vi "Controller Open Synchronization Objects.vi"(8 "error in (no error)":errorcluster, 11 "FOFB Configuration":T4={"FOFB Parameters"={"Network"={"FOFB Controller IP"="", "LNLS Control Network IP"="", "LNLS Control Network Power Supplies TCP Port"=0, "LNLS Control Network FOFB Configuration TCP Port"=0, "LNLS Control Network BPMs TCP Port"=0, "Monitoring Data TCP Port"=0, "Fast Archiver TCP Port"=0, "Fast Command TCP Port"=0, "TCP Listening Timeout"=0}, "Fast Acquisition"={"Sampling Period"=0, "Data Buffer Size"=0, "Monitoring Period"=0}, "Acquisition Network"=[], "Actuation Network"=[]}, "Number of Acquisition Chassis"=0, "Number of Actuation Chassis"=0, "Number of BPM Readings"=0, "BPM Reading Names"=[], "Selected BPM Readings"=[0, 1, 2, 3, 4, 5, 6, 7, 8, 9, 10, 11, 12, 13, 14, 15, 16, 17, 18, 19, 20, 21, 22, 23, 24, 25, 26, 27, 28, 29, 30, 31, 32, 33, 34, 35, 36, 37, 38, 39, 40, 41, 42, 43, 44, 45, 46, 47, 48, 49], "Number of Correctors"=0, "Corrector Names"=[], "Selected Correctors"=[0, 1, 2, 3, 4, 5, 6, 7, 8, 9, 10, 11, 12, 13, 14, 15, 16, 17, 18, 19, 20, 21, 22, 23, 24, 25, 26, 27, 28, 29, 30, 31, 32, 33, 34, 35, 36, 37, 38, 39, 40, 41, 42, 43, 44, 45, 46, 47, 48, 49], "Response Matrix"=[], "Reference Orbit"=[], "Correction Matrix"=[], "FPGA Filter Sets"=[], "Acquisition Chassis Names"=[], "Actuation Chassis Names"=[], "Acquisition Variables"=[], "Actuation Variables"=[], "PS Matrix Mapping"=[], "Inverse PS Matrix Mapping"=[], "BPM Matrix Mapping"=[], "Inverse BPM Matrix Mapping"=[], "BPM Planes"=[], "Corrector Planes"=[]}) -> (0 "error out":errorcluster, 3 "Sync Objects":T1)   [LabVIEW 2011, in "Controller VIs.lvlib"]
uses:
  Controller VIs.lvlib
  Types Definitions/Type FOFB Configuration.ctl
  Types Definitions/Type FOFB Parameters.ctl
  Types Definitions/Type Network Configuration.ctl
  Types Definitions/Type FA Configuration.ctl
  Types Definitions/Type Acquisition Network Configuration.ctl
  Types Definitions/Type Actuation Network Configuration.ctl
  Types Definitions/Type Synchronization Objects.ctl
  Types Definitions/Type Blocking Synchronization Objects.ctl
  Types Definitions/Type Monitoring Data.ctl
  Types Definitions/Type Operation Mode State.ctl
  Types Definitions/Type Diagnostics Data.ctl
  Types Definitions/Type CPU Loads Array.ctl
  Types Definitions/Type CPU Loads.ctl
  Types Definitions/Type Non-blocking Synchronization Objects.ctl
  Types Definitions/Type FOFB Variables.ctl
  Types Definitions/Type Actuation State.ctl
  Type Definitions.lvlib
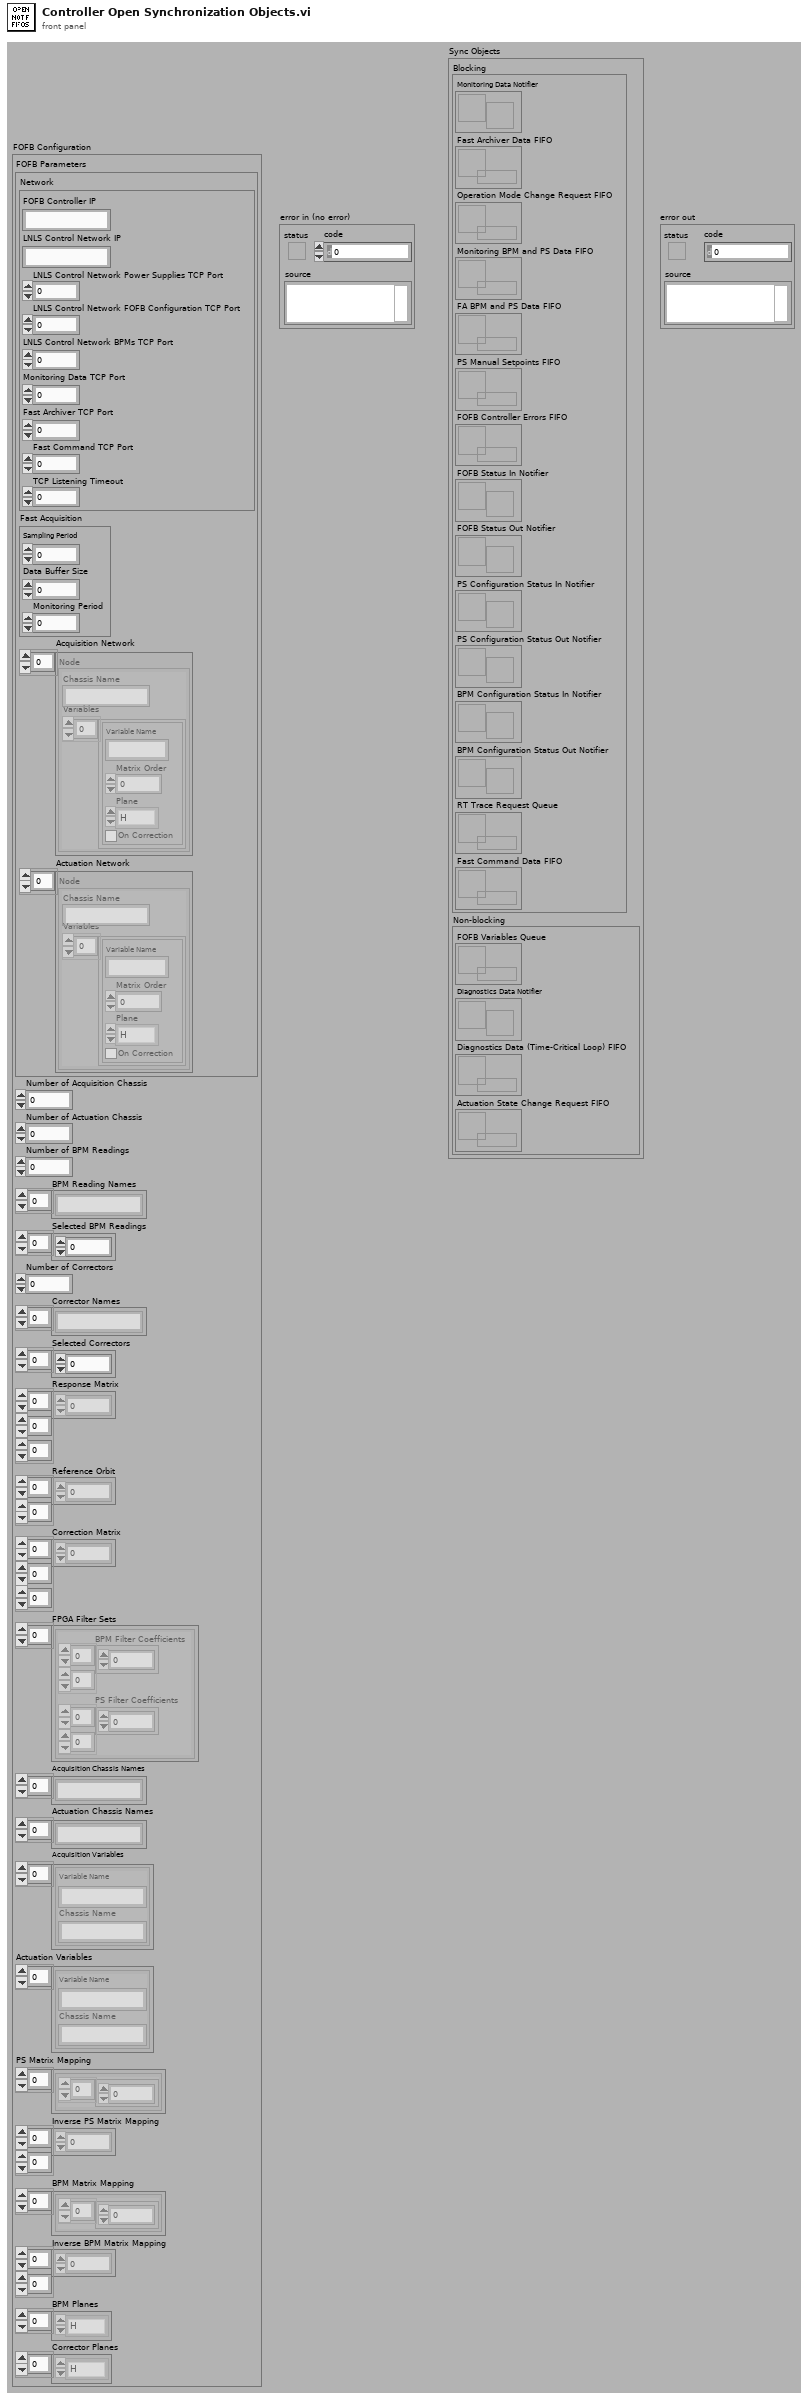
[diagram p1: front panel]
types:
  T1 = typedef "Type Definitions.lvlib/Type Synchronization Objects.ctl" = cluster{"Blocking":T2, "Non-blocking":T3}
  T2 = typedef "Type Definitions.lvlib/Type Blocking Synchronization Objects.ctl" = cluster{"Monitoring Data Notifier":refnum<notifier>, "Fast Archiver Data FIFO":refnum<queue>, "Operation Mode Change Request FIFO":refnum<k33>, "Monitoring BPM and PS Data FIFO":refnum<k33>, "FA BPM and PS Data FIFO":refnum<k33>, "PS Manual Setpoints FIFO":refnum<k33>, "FOFB Controller Errors FIFO ":refnum<k33>, "FOFB Status In Notifier":refnum<notifier>, "FOFB Status Out Notifier":refnum<notifier>, "PS Configuration Status In Notifier":refnum<notifier>, "PS Configuration Status Out Notifier":refnum<notifier>, "BPM Configuration Status In Notifier":refnum<notifier>, "BPM Configuration Status Out Notifier":refnum<notifier>, "RT Trace Request Queue":refnum<queue>, "Fast Command Data FIFO":refnum<k33>}
  T3 = typedef "Type Definitions.lvlib/Type Non-blocking Synchronization Objects.ctl" = cluster{"FOFB Variables Queue":refnum<queue>, "Diagnostics Data Notifier":refnum<notifier>, "Diagnostics Data (Time-Critical Loop) FIFO":refnum<k33>, "Actuation State Change Request FIFO":refnum<k33>}
  T4 = typedef "Type Definitions.lvlib/Type FOFB Configuration.ctl" = cluster{"FOFB Parameters":T5, "Number of Acquisition Chassis":i32, "Number of Actuation Chassis":i32, "Number of BPM Readings":i32, "BPM Reading Names":string[], "Selected BPM Readings":u32[], "Number of Correctors":i32, "Corrector Names":string[], "Selected Correctors":u32[], "Response Matrix":dbl[][][], "Reference Orbit":dbl[][], "Correction Matrix":dbl[][][], "FPGA Filter Sets":cluster{"BPM Filter Coefficients":dbl[][], "PS Filter Coefficients":dbl[][]}[], "Acquisition Chassis Names":string[], "Actuation Chassis Names":string[], "Acquisition Variables":cluster{"Variable Name":string, "Chassis Name":string}[], "Actuation Variables":cluster{"Variable Name":string, "Chassis Name":string}[], "PS Matrix Mapping":cluster{u32[]}[], "Inverse PS Matrix Mapping":u32[][], "BPM Matrix Mapping":cluster{u32[]}[], "Inverse BPM Matrix Mapping":u32[][], "BPM Planes":enum8{"H", "V"}[], "Corrector Planes":enum8{"H", "V"}[]}
  T5 = typedef "Type Definitions.lvlib/Type FOFB Parameters.ctl" = cluster{"Network":T6, "Fast Acquisition":T7, "Acquisition Network":T8, "Actuation Network":T9}
  T6 = typedef "Type Definitions.lvlib/Type Network Configuration.ctl" = cluster{"FOFB Controller IP":string, "LNLS Control Network IP":string, "LNLS Control Network Power Supplies TCP Port":u16, "LNLS Control Network FOFB Configuration TCP Port":u16, "LNLS Control Network BPMs TCP Port":u16, "Monitoring Data TCP Port":u16, "Fast Archiver TCP Port":u16, "Fast Command TCP Port":u16, "TCP Listening Timeout":i32}
  T7 = typedef "Type Definitions.lvlib/Type FA Configuration.ctl" = cluster{"Sampling Period":u32, "Data Buffer Size":u32, "Monitoring Period":u32}
  T8 = typedef "Type Definitions.lvlib/Type Acquisition Network Configuration.ctl" = cluster{"Chassis Name":string, "Variables":cluster{"Variable Name":string, "Matrix Order":u32, "Plane":enum8{"H", "V"}, "On Correction":bool}[]}[]
  T9 = typedef "Type Definitions.lvlib/Type Actuation Network Configuration.ctl" = cluster{"Chassis Name":string, "Variables":cluster{"Variable Name":string, "Matrix Order":u32, "Plane":enum8{"H", "V"}, "On Correction":bool}[]}[]
  T10 = typedef "Type Definitions.lvlib/Type Operation Mode State.ctl" = enum8{"Idle Mode", "Manual Mode", "FOFB Mode"}
  T11 = typedef "Type Definitions.lvlib/Type FOFB Variables.ctl" = cluster{"Reference Orbit":dbl[], "Response Matrix":dbl[][], "Correction Matrix":dbl[][], "FPGA Filter":cluster{"BPM Filter Coefficients":dbl[][], "PS Filter Coefficients":dbl[][]}, "Selected BPM Readings":u32[], "Selected Correctors":u32[], "BPM Planes":enum8{"H", "V"}[], "Corrector Planes":enum8{"H", "V"}[], "Fast Command Enabled":bool, "Horizontal Gain":dbl, "Vertical Gain":dbl, "Horizontal Distortion Threshold":dbl, "Vertical Distortion Threshold":dbl}
  T12 = cluster{"read mode":enum16{"polling", "blocking"}, "write mode":enum16{"polling", "blocking"}}
  T13 = typedef "Type Definitions.lvlib/Type Diagnostics Data.ctl" = cluster{"Time-Critical Loop Missed Iterations":u32, "Time-Critical Loop Execution Time (usec)":u32, "Available Memory (bytes)":u32, "CPU Loads Array":T14}
  T14 = typedef "Type Definitions.lvlib/Type CPU Loads Array.ctl" = T15[]
  T15 = typedef "Type Definitions.lvlib/Type CPU Loads.ctl" = cluster{"Total (%)":dbl, "Time Critical (%)":dbl, "Timed Structures (%)":dbl, "High (%)":dbl, "Above Normal (%)":dbl, "Normal (%)":dbl, "Background (%)":dbl, "Idle (%)":dbl, "ISR (%)":dbl}
  T16 = typedef "Type Definitions.lvlib/Type Monitoring Data.ctl" = cluster{"Timestamp":timestamp, "BPM Readings":dbl[], "PS Readings":dbl[], "PS FOFB Setpoints":dbl[], "PS Status per Rack":u8[], "PS ON-OFF per Rack":u8[], "Operation Mode":T10, "Diagnostics Data":T13, "Controller Status Table":i32[]}
  T17 = typedef "Type Definitions.lvlib/Type Actuation State.ctl" = enum8{"Only reading", "Manual", "FOFB Initialization", "FOFB", "FOFB Stopping"}
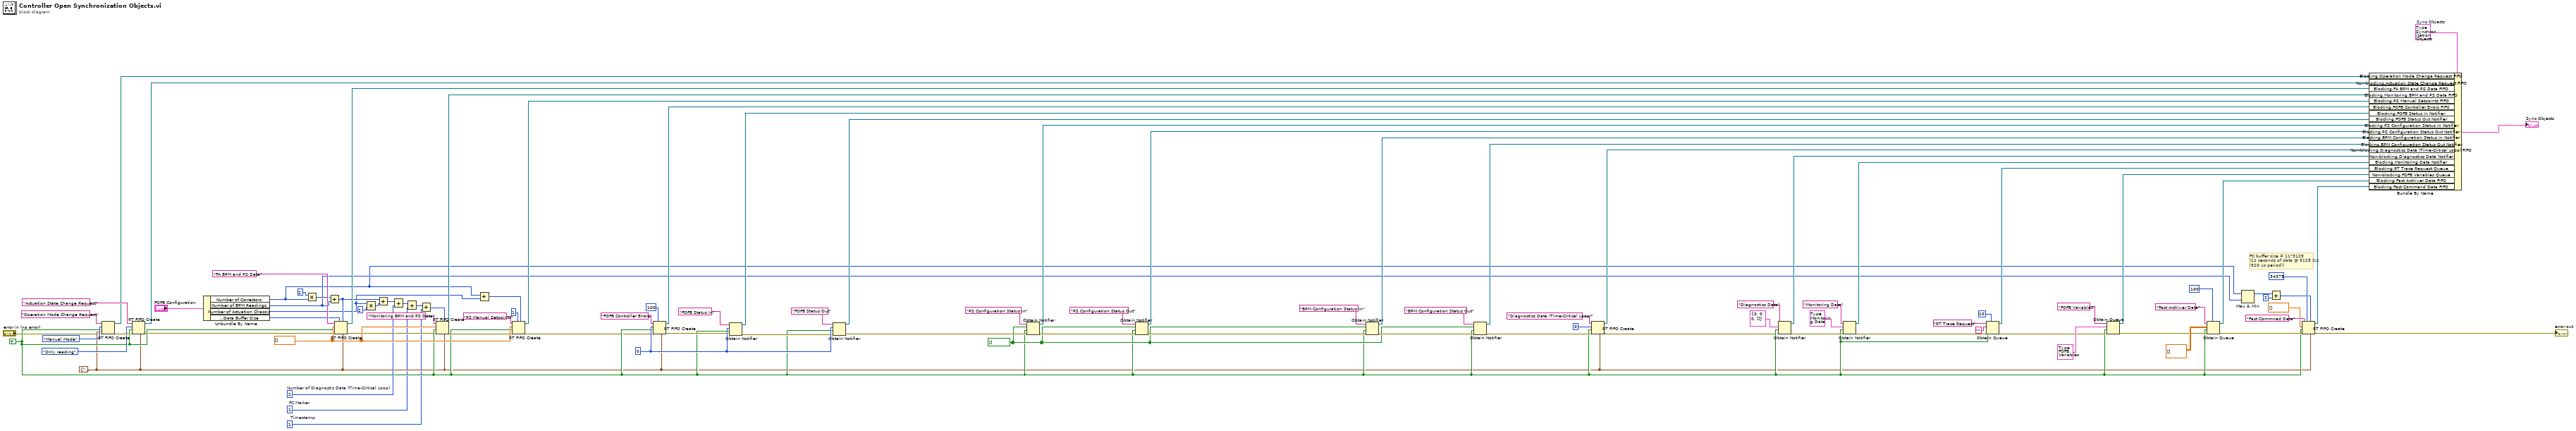
[diagram p0: block diagram]
diagram:
  w5 = 1  # FC Marker
  w4 = 1  # Timestamp
  w30 = bool[] []
  w64 = 2  # Number of Diagnostic Data (Time-Critical Loop)
  w14 = T12 {"read mode"=enum."blocking", "write mode"=enum."blocking"} ("r/w modes (polling,polling)")
  w41 = u16 0 ("elements in array (1)")
  w97 = T1 {"Blocking"={"Monitoring Data Notifier"=refnum, "Fast Archiver Data FIFO"=refnum, "Operation Mode Change Request FIFO"=refnum, "Monitoring BPM and PS Data FIFO"=refnum, "FA BPM and PS Data FIFO"=refnum, "PS Manual Setpoints FIFO"=refnum, "FOFB Controller Errors FIFO "=refnum, "FOFB Status In Notifier"=refnum, "FOFB Status Out Notifier"=refnum, "PS Configuration Status In Notifier"=refnum, "PS Configuration Status Out Notifier"=refnum, "BPM Configuration Status In Notifier"=refnum, "BPM Configuration Status Out Notifier"=refnum, "RT Trace Request Queue"=refnum, "Fast Command Data FIFO"=refnum}, "Non-blocking"={"FOFB Variables Queue"=refnum, "Diagnostics Data Notifier"=refnum, "Diagnostics Data (Time-Critical Loop) FIFO"=refnum, "Actuation State Change Request FIFO"=refnum}}  # Sync Objects
  w20 = TRUE
  w74 = dbl[] [] ("BPM Readings")
  # "FC buffer size = 11*3125\n(11 seconds of data @ 3125 S/s\n(320 us period))"
  n1 = RT FIFO Create(0:"Operation Mode Change Request" ("name (unnamed)"), 1:Type_Operation_Mode_State."Manual Mode" ("Operation Mode"), 2:w20, 3:"error in (no error)", 7:w14) -> (8:w54:refnum<k33>, 11:w94:errorcluster)  [unwired: 3 in, 1 out]
  n2 = RT FIFO Create(0:"Actuation State Change Request" ("name (unnamed)"), 1:Type_Actuation_State."Only reading" ("Actuation State"), 2:w20, 3:w94, 7:w14) -> (8:w89:refnum<k33>, 11:w9:errorcluster)  [unwired: 3 in, 1 out]
  n3 = Unbundle By Name("FOFB Configuration") -> ("Number of Correctors"=w19:i32, "Number of BPM Readings"=w21:i32, "Number of Actuation Chassis"=w18:i32, "FOFB Parameters.Fast Acquisition.Data Buffer Size"=w84:u32)
  n4 = Multiply(x=2 ("y"), y=w19) -> (x*y=w85:i32)
  n5 = Add(x=w85, y=w21) -> (x+y=w78:i32)
  n6 = RT FIFO Create(0:"FA BPM and PS Data" ("name (unnamed)"), 1:w74, 2:w20, 3:w9, 4:w84, 6:w78, 7:w14) -> (8:w98:refnum<k33>, 11:w10:errorcluster)  [unwired: 1 in, 1 out]
  n7 = Multiply(x=w18, y=2) -> (x*y=w70:i32)
  n8 = Add(x=w78, y=w70) -> (x+y=w65:i32)
  n9 = Add(x=w65, y=w64) -> (x+y=w7:i32)
  n10 = Add(x=w7, y=w5) -> (x+y=w6:i32)
  n11 = Add(x=w6, y=w4) -> (x+y=w8:i32)
  n12 = RT FIFO Create(0:"Monitoring BPM and PS Data" ("name (unnamed)"), 1:w74, 2:w20, 3:w10, 6:w8, 7:w14) -> (8:w87:refnum<k33>, 11:w73:errorcluster)  [unwired: 2 in, 1 out]
  n13 = Add(x=w19, y=w18) -> (x+y=w72:i32)
  n14 = RT FIFO Create(0:"PS Manual Setpoints" ("name (unnamed)"), 1:w74, 2:w20, 3:w73, 4:u32 1 ("size (10)"), 6:w72) -> (8:w71:refnum<k33>, 11:w13:errorcluster)  [unwired: 2 in, 1 out]
  n15 = RT FIFO Create(0:"FOFB Controller Errors" ("name (unnamed)"), 1:w41, 2:w20, 3:w13, 4:u32 100 ("elements in array (1)"), 7:w14) -> (8:w52:refnum<k33>, 11:w38:errorcluster)  [unwired: 2 in, 1 out]
  n16 = Obtain Notifier(name (unnamed)="FOFB Status In", notification data type=w41, create if not found? (T)=w20, error in (no error)=w38) -> (notifier out=w39:refnum<notifier>, error out=w37:errorcluster)  [unwired: 1 out]
  n17 = Obtain Notifier(name (unnamed)="FOFB Status Out", notification data type=w41, create if not found? (T)=w20, error in (no error)=w37) -> (notifier out=w40:refnum<notifier>, error out=w32:errorcluster)  [unwired: 1 out]
  n18 = Obtain Notifier(name (unnamed)="PS Configuration Status In", notification data type=w30, create if not found? (T)=w20, error in (no error)=w32) -> (notifier out=w36:refnum<notifier>, error out=w50:errorcluster)  [unwired: 1 out]
  n19 = Obtain Notifier(name (unnamed)="PS Configuration Status Out", notification data type=w30, create if not found? (T)=w20, error in (no error)=w50) -> (notifier out=w35:refnum<notifier>, error out=w31:errorcluster)  [unwired: 1 out]
  n20 = Obtain Notifier(name (unnamed)="BPM Configuration Status In", notification data type=w30, create if not found? (T)=w20, error in (no error)=w31) -> (notifier out=w34:refnum<notifier>, error out=w45:errorcluster)  [unwired: 1 out]
  n21 = Obtain Notifier(name (unnamed)="BPM Configuration Status Out", notification data type=w30, create if not found? (T)=w20, error in (no error)=w45) -> (notifier out=w33:refnum<notifier>, error out=w44:errorcluster)  [unwired: 1 out]
  n22 = RT FIFO Create(0:"Diagnostics Data (Time-Critical Loop)" ("name (unnamed)"), 1:u32 0 ("elements in array (1)"), 2:w20, 3:w44, 7:w14) -> (8:w66:refnum<k33>, 11:w12:errorcluster)  [unwired: 3 in, 1 out]
  n23 = Obtain Notifier(name (unnamed)="Diagnostics Data", notification data type=T13 {"Time-Critical Loop Missed Iterations"=0, "Time-Critical Loop Execution Time (usec)"=0, "Available Memory (bytes)"=0, "CPU Loads Array"=[]} ("Diagnostics Data"), create if not found? (T)=w20, error in (no error)=w12) -> (notifier out=w79:refnum<notifier>, error out=w80:errorcluster)  [unwired: 1 out]
  n24 = Obtain Notifier(name (unnamed)="Monitoring Data", notification data type=T16 {"Timestamp"=timestamp(0 s since 1904-01-01), "BPM Readings"=[], "PS Readings"=[], "PS FOFB Setpoints"=[], "PS Status per Rack"=[], "PS ON-OFF per Rack"=[], "Operation Mode"=enum."Idle Mode", "Diagnostics Data"={"Time-Critical Loop Missed Iterations"=0, "Time-Critical Loop Execution Time (usec)"=0, "Available Memory (bytes)"=0, "CPU Loads Array"=[]}, "Controller Status Table"=[]} ("Slow Data"), create if not found? (T)=w20, error in (no error)=w80) -> (notifier out=w91:refnum<notifier>, error out=w58:errorcluster)  [unwired: 1 out]
  n25 = Obtain Queue(max queue size (-1, unlimited)=10, name (unnamed)="RT Trace Request", element data type="" ("Host IP Address"), create if not found? (T)=w20, error in (no error)=w58) -> (queue out=w55:refnum<queue>, error out=w57:errorcluster)  [unwired: 1 out]
  n26 = Obtain Queue(name (unnamed)="FOFB Variables", element data type=T11 {"Reference Orbit"=[], "Response Matrix"=[], "Correction Matrix"=[], "FPGA Filter"={"BPM Filter Coefficients"=[], "PS Filter Coefficients"=[]}, "Selected BPM Readings"=[], "Selected Correctors"=[], "BPM Planes"=[], "Corrector Planes"=[], "Fast Command Enabled"=FALSE, "Horizontal Gain"=0.0, "Vertical Gain"=0.0, "Horizontal Distortion Threshold"=0.0, "Vertical Distortion Threshold"=0.0} ("FOFB Variables 2"), create if not found? (T)=w20, error in (no error)=w57) -> (queue out=w61:refnum<queue>, error out=w26:errorcluster)  [unwired: 1 in, 1 out]
  n27 = Obtain Queue(max queue size (-1, unlimited)=100, name (unnamed)="Fast Archiver Data", element data type=sgl[][] [] ("BPM Readings"), create if not found? (T)=w20, error in (no error)=w26) -> (queue out=w25:refnum<queue>, error out=w22:errorcluster)  [unwired: 1 out]
  n28 = Max & Min(x=w19, y=w21) -> (max(x,y)=w3:i32)  [unwired: 1 out]
  n29 = Add(x=w3, y=2) -> (x+y=w2:i32)
  n30 = RT FIFO Create(0:"Fast Commnad Data" ("name (unnamed)"), 1:sgl[] [], 2:w20, 3:w22, 4:u32 34375 ("datapoints in waveform (1)"), 6:w2, 7:w14) -> (8:w16:refnum<k33>, 11:→"error out":errorcluster)  [unwired: 1 in, 1 out]
  n31 = Bundle By Name(cluster=w97, "Blocking.Operation Mode Change Request FIFO"=w54, "Non-blocking.Actuation State Change Request FIFO"=w89, "Blocking.FA BPM and PS Data FIFO"=w98, "Blocking.Monitoring BPM and PS Data FIFO"=w87, "Blocking.PS Manual Setpoints FIFO"=w71, "Blocking.FOFB Controller Errors FIFO"=w52, "Blocking.FOFB Status In Notifier"=w39, "Blocking.FOFB Status Out Notifier"=w40, "Blocking.PS Configuration Status In Notifier"=w36, "Blocking.PS Configuration Status Out Notifier"=w35, "Blocking.BPM Configuration Status In Notifier"=w34, "Blocking.BPM Configuration Status Out Notifier"=w33, "Non-blocking.Diagnostics Data (Time-Critical Loop) FIFO"=w66, "Non-blocking.Diagnostics Data Notifier"=w79, "Blocking.Monitoring Data Notifier"=w91, "Blocking.RT Trace Request Queue"=w55, "Non-blocking.FOFB Variables Queue"=w61, "Blocking.Fast Archiver Data FIFO"=w25, "Blocking.Fast Command Data FIFO"=w16) -> (→"Sync Objects":T1)
